vi "VariableCheck.vi"(8 "error in (no error)":errorcluster, 9 "OriginalName":string, 10 "VariableIn":refnum<class "Variable.lvclass">, 11 "VariableManager in":refnum<class "VariableManager.lvclass">) -> (0 "error out":errorcluster, 1 "RejectMessage":string, 2 "Pass":bool=TRUE, 3 "VariableManager out":refnum<class "VariableManager.lvclass">)   [LabVIEW 2013, in "VariableManager.lvclass"]
doc: "Check the given variable definition before adding to database.\n\nReturn true if the given variable passes all tests.\nReturn false if the given variable fails some tests.\nRejectMessage can be used to identify the failed tests.\n\nThe following will make a variable definition fails the test:\n1. The difinition has an empty name\n2. The variable is set to be sequenced but the sequence function is not specified.\n3. The name is already used by another sequence index.\n4. The name is already used by another variable. Providing OriginalName will bypass the check against the given OriginalName\n5. The name begins with number.\n6. The name is reserved (GlobalReservedNames.vi)"
uses:
  VariableManager.lvclass
  Variable/Variable.lvclass
  GlobalReservedNames.vi
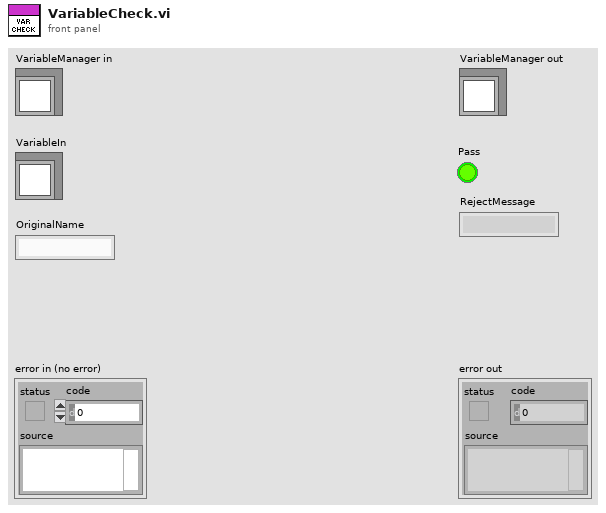
[diagram p1: front panel]
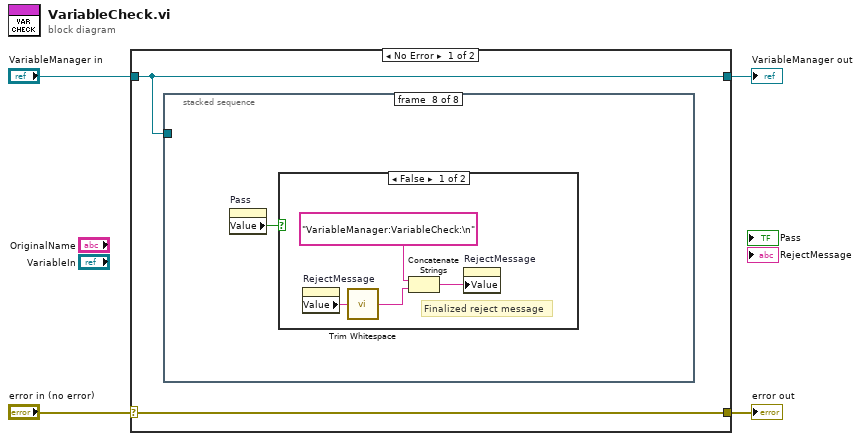
[diagram p0: block diagram]
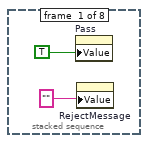
[diagram p2: hidden frame]
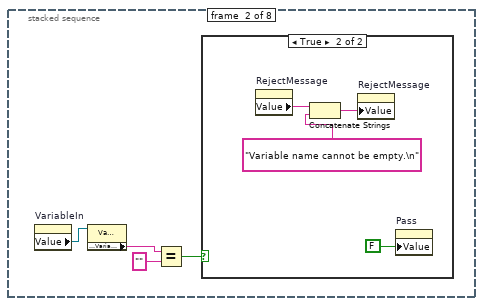
[diagram p3: hidden frame]
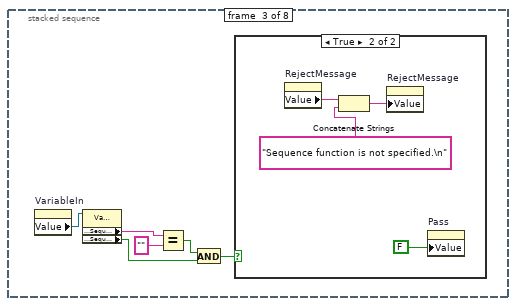
[diagram p5: hidden frame]
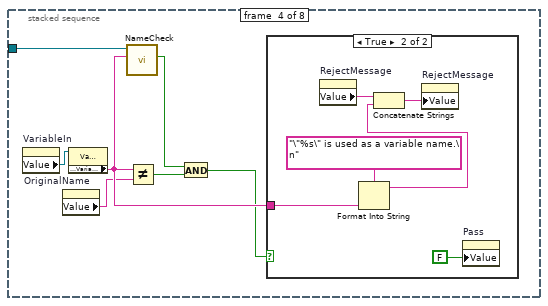
[diagram p7: hidden frame]
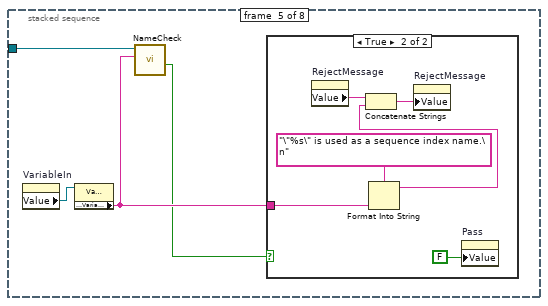
[diagram p9: hidden frame]
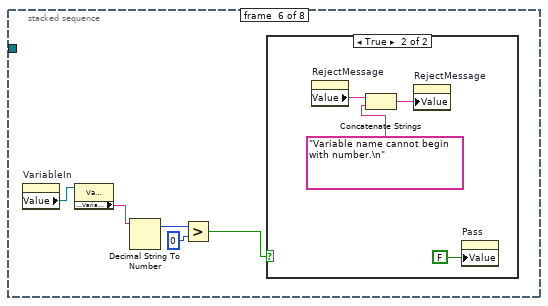
[diagram p11: hidden frame]
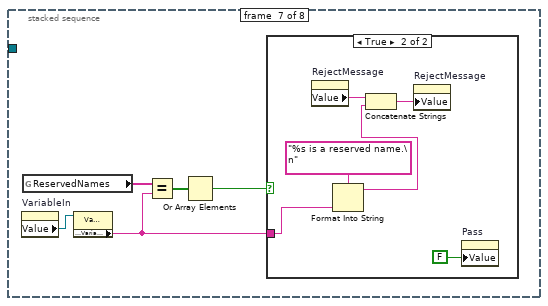
[diagram p13: hidden frame]
diagram:
  n1 = case shown="No Error" "error in (no error)" {
    selector: "error in (no error)" -> [w6 w76]
    tunnel: [w6 w76] -> w3
    tunnel: [w5 w75] -> w1
    tunnel: "VariableManager in" -> [w5 w75]
    frame No Error {
      n2 = stacked-sequence {
        tunnel: w5 -> [_ _ _ w27 w40 _ _ _]
        frame #0 {
          n3 = property on="Pass" class="Bool (strict)"("Value"=TRUE ("Pass")) -> ()  [unwired: 2 in, 2 out]
          n4 = property on="RejectMessage" class="Str"("Value"="") -> ()  [unwired: 2 in, 2 out]
        }
        frame #1 {
          n5 = property on="VariableIn" class="LVClassControl (strict)"() -> ("Value"=w10:refnum<class "Variable.lvclass">)  [unwired: 2 in, 2 out]
          n6 = property class="Variable.lvclass"(reference=w10) -> ("Accessors:VariableName"=w12:string)  [unwired: 1 in, 2 out]
          n7 = Equal?(x=w12, y="") -> (x = y?=w9:bool)
          n8 = case shown="True" w9 {
            frame False {
            }
            frame True {
              n9 = property on="RejectMessage" class="Str"() -> ("Value"=w15:string)  [unwired: 2 in, 2 out]
              n10 = Concatenate Strings(w15, "Variable name cannot be empty.\n") -> (w14:string)
              n11 = property on="RejectMessage" class="Str"("Value"=w14) -> ()  [unwired: 2 in, 2 out]
              n12 = property on="Pass" class="Bool (strict)"("Value"=FALSE ("Pass")) -> ()  [unwired: 2 in, 2 out]
            }
          }
        }
        frame #2 {
          n13 = property on="VariableIn" class="LVClassControl (strict)"() -> ("Value"=w18:refnum<class "Variable.lvclass">)  [unwired: 2 in, 2 out]
          n14 = property class="Variable.lvclass"(reference=w18) -> ("Accessors:SequenceFunction"=w22:string, "Accessors:Sequence"=w20:bool)  [unwired: 1 in, 2 out]
          n15 = Equal?(x=w22, y="") -> (x = y?=w19:bool)
          n16 = And(x=w19, y=w20) -> (x .and. y?=w17:bool)
          n17 = case shown="True" w17 {
            frame False {
            }
            frame True {
              n18 = property on="RejectMessage" class="Str"() -> ("Value"=w25:string)  [unwired: 2 in, 2 out]
              n19 = Concatenate Strings(w25, "Sequence function is not specified.\n") -> (w24:string)
              n20 = property on="RejectMessage" class="Str"("Value"=w24) -> ()  [unwired: 2 in, 2 out]
              n21 = property on="Pass" class="Bool (strict)"("Value"=FALSE ("Pass")) -> ()  [unwired: 2 in, 2 out]
            }
          }
        }
        frame #3 {
          n22 = property on="VariableIn" class="LVClassControl (strict)"() -> ("Value"=w29:refnum<class "Variable.lvclass">)  [unwired: 2 in, 2 out]
          n23 = property on="OriginalName" class="Str"() -> ("Value"=w30:string)  [unwired: 2 in, 2 out]
          n24 = property class="Variable.lvclass"(reference=w29) -> ("Accessors:VariableName"=w32:string)  [unwired: 1 in, 2 out]
          n25 = call-dynamic "NameCheck.vi"("Name"=w32, "VariableManager in"=w27) -> ("UsedAsVariable"=w31:bool)  [unwired: 6 in, 3 out]
          n26 = Not Equal?(x=w32, y=w30) -> (x != y?=w33:bool)
          n27 = And(x=w31, y=w33) -> (x .and. y?=w28:bool)
          n28 = case shown="True" w28 {
            tunnel: w32 -> [_ w39]
            frame False {
            }
            frame True {
              n29 = property on="RejectMessage" class="Str"() -> ("Value"=w36:string)  [unwired: 2 in, 2 out]
              n30 = Format Into String(format string="\"%s\" is used as a variable name.\n", w39) -> (resulting string=w34:string)  [unwired: 2 in, 1 out]
              n31 = Concatenate Strings(w36, w34) -> (w35:string)
              n32 = property on="RejectMessage" class="Str"("Value"=w35) -> ()  [unwired: 2 in, 2 out]
              n33 = property on="Pass" class="Bool (strict)"("Value"=FALSE ("Pass")) -> ()  [unwired: 2 in, 2 out]
            }
          }
        }
        frame #4 {
          n34 = property on="VariableIn" class="LVClassControl (strict)"() -> ("Value"=w42:refnum<class "Variable.lvclass">)  [unwired: 2 in, 2 out]
          n35 = property class="Variable.lvclass"(reference=w42) -> ("Accessors:VariableName"=w43:string)  [unwired: 1 in, 2 out]
          n36 = call-dynamic "NameCheck.vi"("Name"=w43, "VariableManager in"=w40) -> ("UsedAsSequenceIndex"=w41:bool)  [unwired: 6 in, 3 out]
          n37 = case shown="True" w41 {
            tunnel: w43 -> [_ w49]
            frame False {
            }
            frame True {
              n38 = property on="RejectMessage" class="Str"() -> ("Value"=w46:string)  [unwired: 2 in, 2 out]
              n39 = Format Into String(format string="\"%s\" is used as a sequence index name.\n", w49) -> (resulting string=w44:string)  [unwired: 2 in, 1 out]
              n40 = Concatenate Strings(w46, w44) -> (w45:string)
              n41 = property on="RejectMessage" class="Str"("Value"=w45) -> ()  [unwired: 2 in, 2 out]
              n42 = property on="Pass" class="Bool (strict)"("Value"=FALSE ("Pass")) -> ()  [unwired: 2 in, 2 out]
            }
          }
        }
        frame #5 {
          n43 = property on="VariableIn" class="LVClassControl (strict)"() -> ("Value"=w54:refnum<class "Variable.lvclass">)  [unwired: 2 in, 2 out]
          n44 = property class="Variable.lvclass"(reference=w54) -> ("Accessors:VariableName"=w53:string)  [unwired: 1 in, 2 out]
          n45 = Decimal String To Number(string=w53) -> (offset past number=w52:i32)  [unwired: 2 in, 1 out]
          n46 = Greater?(x=w52, y=0) -> (0:w50:bool)
          n47 = case shown="True" w50 {
            frame False {
            }
            frame True {
              n48 = property on="RejectMessage" class="Str"() -> ("Value"=w57:string)  [unwired: 2 in, 2 out]
              n49 = Concatenate Strings(w57, "Variable name cannot begin with number.\n") -> (w56:string)
              n50 = property on="RejectMessage" class="Str"("Value"=w56) -> ()  [unwired: 2 in, 2 out]
              n51 = property on="Pass" class="Bool (strict)"("Value"=FALSE ("Pass")) -> ()  [unwired: 2 in, 2 out]
            }
          }
        }
        frame #6 {
          n52 = property on="VariableIn" class="LVClassControl (strict)"() -> ("Value"=w63:refnum<class "Variable.lvclass">)  [unwired: 2 in, 2 out]
          n53 = global read "GlobalReservedNames.vi" "ReservedNames"() -> (w62:string[])
          n54 = property class="Variable.lvclass"(reference=w63) -> ("Accessors:VariableName"=w59:string)  [unwired: 1 in, 2 out]
          n55 = Equal?(x=w62, y=w59) -> (x = y?=w61:bool[])
          n56 = Or Array Elements(Boolean array=w61) -> (logical OR=w60:bool)
          n57 = case shown="True" w60 {
            tunnel: w59 -> [_ w64]
            frame False {
            }
            frame True {
              n58 = property on="RejectMessage" class="Str"() -> ("Value"=w68:string)  [unwired: 2 in, 2 out]
              n59 = Format Into String(format string="%s is a reserved name.\n", w64) -> (resulting string=w65:string)  [unwired: 2 in, 1 out]
              n60 = Concatenate Strings(w68, w65) -> (w67:string)
              n61 = property on="RejectMessage" class="Str"("Value"=w67) -> ()  [unwired: 2 in, 2 out]
              n62 = property on="Pass" class="Bool (strict)"("Value"=FALSE ("Pass")) -> ()  [unwired: 2 in, 2 out]
            }
          }
        }
        frame #7 {
          n63 = property on="Pass" class="Bool (strict)"() -> ("Value"=w70:bool)  [unwired: 2 in, 2 out]
          n64 = case shown="False" w70 {
            frame False {
              # "Finalized reject message"
              n65 = property on="RejectMessage" class="Str"() -> ("Value"=w74:string)  [unwired: 2 in, 2 out]
              n66 = call <vilib>:"Trim Whitespace.vi"("string"=w74) -> ("trimmed string"=w72:string)  [unwired: 1 in]
              n67 = Concatenate Strings("VariableManager:VariableCheck:\n", w72) -> (w71:string)
              n68 = property on="RejectMessage" class="Str"("Value"=w71) -> ()  [unwired: 2 in, 2 out]
            }
            frame True {
            }
          }
        }
      }
    }
    frame Error {
    }
  }
  "error out" <- w3
  "VariableManager out" <- w1
